vi "Go to Speed.vi"(6 "Max RPM Value (MXRPM)":dbl=1000.0, 8 "error in (no error)":errorcluster, 9 "Channel":u8=1, 10 "Speed, RPM":dbl, 11 "VISA resource name":refnum<visa-resource-name>) -> (0 "error out":errorcluster, 2 "Sent Command":string, 3 "VISA resource name out":refnum<visa-resource-name>)   [LabVIEW 2017, in "Roboteq Controller KBL1xxx.lvlib"]
uses:
  <instrlib>/Roboteq Controller KBL1xxx/Roboteq Controller KBL1xxx.lvlib
  <instrlib>/Roboteq Controller KBL1xxx/Private/Support/Command Create (2 parameters).vi
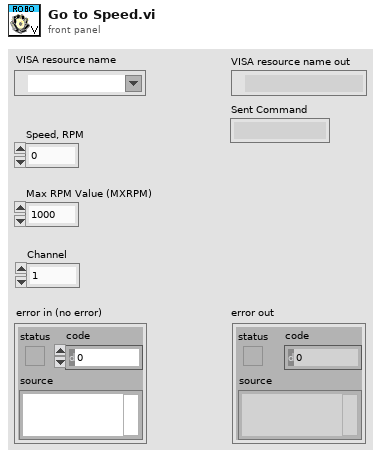
[diagram p1: front panel]
types:
  T1 = enum16{"Runtime", "Configuration", "Maintenance"}
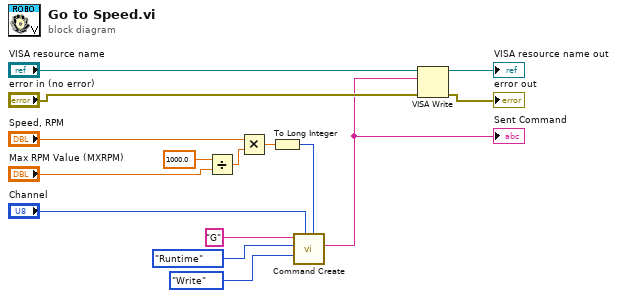
[diagram p0: block diagram]
diagram:
  n1 = Divide(x=1000.0, y="Max RPM Value (MXRPM)") -> (x/y=w12:dbl)
  n2 = Multiply(x="Speed, RPM", y=w12) -> (x*y=w11:dbl)
  n3 = To Long Integer(number=w11) -> (32bit integer=w6:i32)
  n4 = call-poly <instrlib>:"Command Create.vi"("Parameter 2"=w6, "Parameter 1"="Channel", "Command Mode"=enum16{"Write", "Read"}."Write", "Command Type"=T1."Runtime", "Command Name"="G") -> ("Command"=w3:string)  [unwired: 6 in]
  "Sent Command" <- w3
  n5 = VISA Write(VISA resource name="VISA resource name", write buffer=w3, error in (no error)="error in (no error)") -> (VISA resource name out=→"VISA resource name out":refnum<visa-resource-name>, error out=→"error out":errorcluster)  [unwired: 1 out]
